vi "Inficon Hot Density Calculation.vi"(8 "Error In":errorcluster, 11 "RTD Out (°F)":dbl format="%#.6g") -> (0 "Error Out":errorcluster, 3 "Density (lb/gal)":dbl format="%#.6g")   [LabVIEW 2019]
panel:
  out "Upper6":dbl format="%#.6g"
  out "Upper5":dbl format="%#.6g"
  out "Upper4":dbl format="%#.6g"
  out "Upper3":dbl format="%#.6g"
  out "Upper2":dbl format="%#.6g"
  out "Upper1":dbl format="%#.6g"
  out "Lower":dbl format="%#.6g"
  out "Upper":dbl format="%#.6g"
  out "RTDK":dbl format="%.6g"
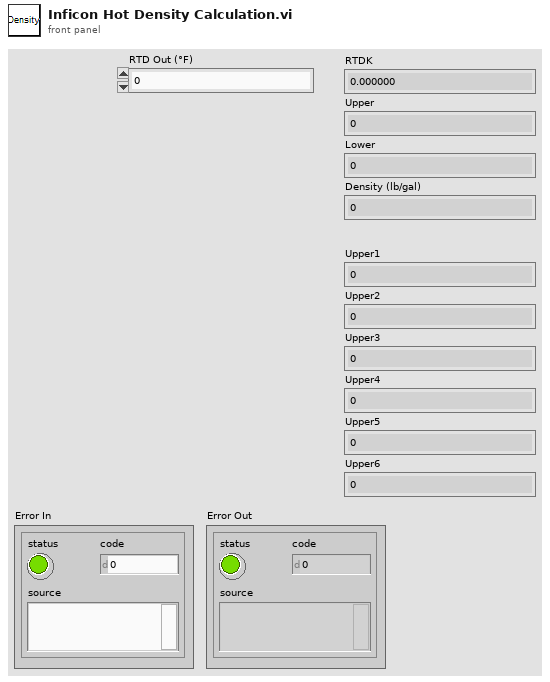
[diagram p1: front panel]
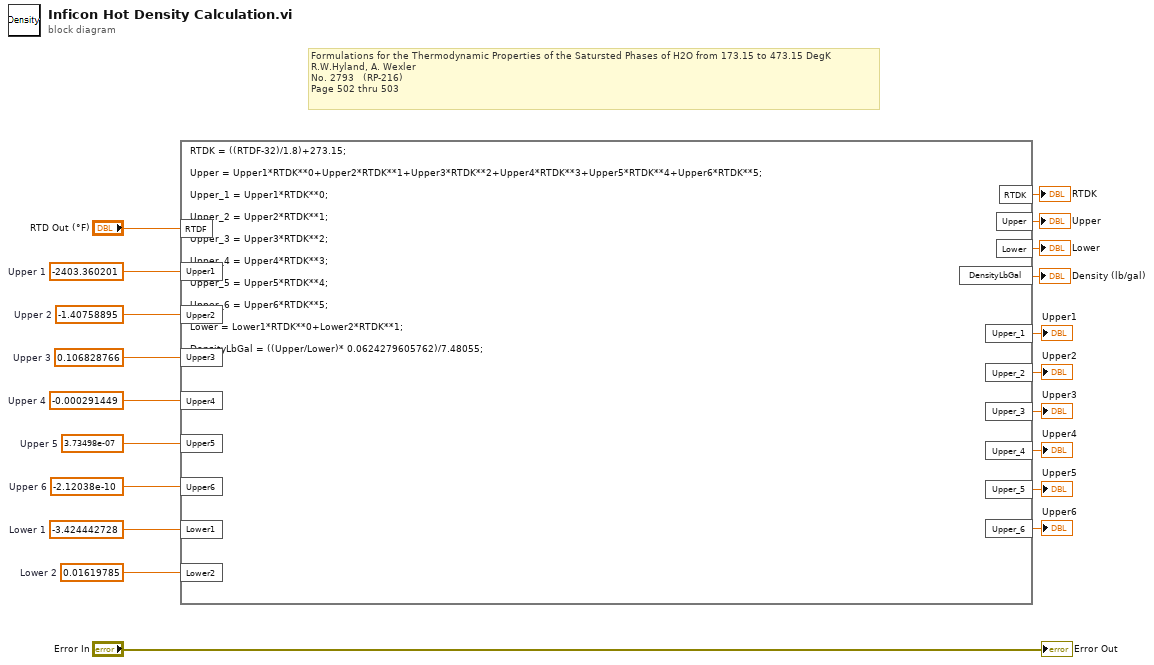
[diagram p0: block diagram]
diagram:
  w11 = 0.01619785  # Lower 2
  w10 = -3.424442728  # Lower 1
  w13 = -2.12038e-10  # Upper 6
  w14 = 3.73498e-07  # Upper 5
  w15 = -0.000291449  # Upper 4
  w16 = 0.106828766  # Upper 3
  w17 = -1.40758895  # Upper 2
  w18 = -2403.360201  # Upper 1
  # "Formulations for the Thermodynamic Properties of the Satursted Phases of H2O from 173.15 to 473.15 DegK\nR.W.Hyland, A. Wexler\nNo. 2793   (RP-216)\nPage 502 thru 503"
  n1 = formula code="RTDK = ((RTDF-32)/1.8)+273.15;\n\nUpper = Upper1*RTDK**0+Upper2*RTDK**1+Upper3*RTDK**2+Upper4*RTDK**3+Upper5*RTDK**4+Upper6*RTDK**5;\n\nUpper_1 = Upper1*RTDK**0;\n\nUpper_2 = Upper2*RTDK**1;\n\nUpper_3 = Upper3*RTDK**2;\n\nUpper_4 = Upper4*RTDK**3;\n\nUpper_5 = Upper5*RTDK**4;\n\nUpper_6 = Upper6*RTDK**5;\n\nLower = Lower1*RTDK**0+Lower2*RTDK**1;\n\nDensityLbGal = ((Upper/Lower)* 0.0624279605762)/7.48055;"("RTDF"="RTD Out (°F)", "Upper1"=w18, "Upper2"=w17, "Upper3"=w16, "Upper4"=w15, "Upper5"=w14, "Upper6"=w13, "Lower1"=w10, "Lower2"=w11) -> ("RTDK"=→"RTDK":dbl, "Upper"=→"Upper":dbl, "Lower"=→"Lower":dbl, "DensityLbGal"=→"Density (lb/gal)":dbl, "Upper_1"=→"Upper1":dbl, "Upper_2"=→"Upper2":dbl, "Upper_3"=→"Upper3":dbl, "Upper_4"=→"Upper4":dbl, "Upper_5"=→"Upper5":dbl, "Upper_6"=→"Upper6":dbl)
  "Error Out" <- "Error In"
